vi "Seg1_Charging_Limit_current.vi"(0 "VISA Refnum in":refnum<visa-resource-name>, 1 "Value":string, 3 "Data Log Period (0.1 s)":dbl=1.0 format="%#_13g", 5 "Set Voltge(V)":dbl=4.35 format="%_3f", 7 "Log?":bool, 9 "Charge Current (A)":dbl=0.06 format="%#_13g", 11 "error in (no error)":errorcluster {"code" format="%.0x"}, 12 "Numeric":i32, 14 "Number of cycles":i32) -> (4 "VISA Refnum out":refnum<visa-resource-name>, 6 "String":string, 8 "File Name Out":string, 10 "String 2":string, 15 "error out":errorcluster)   [LabVIEW 2015]
uses:
  <instrlib>/Agilent N6700 Series/Agilent N6700 Series.lvlib
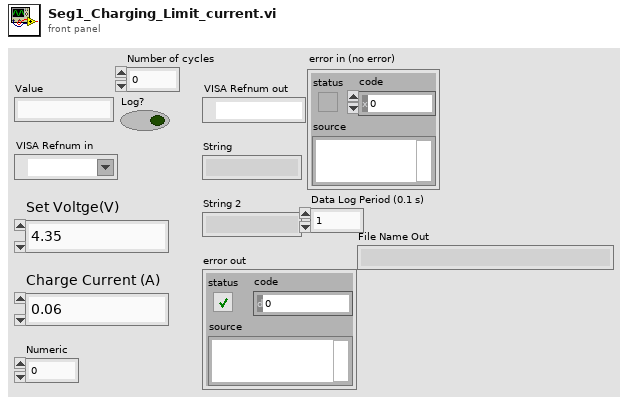
[diagram p1: front panel]
types:
  T1 = enum16{"2 Quad Power Supply", "Unipower Supply", "CC Load", "CV Load", "VM", "CM"}
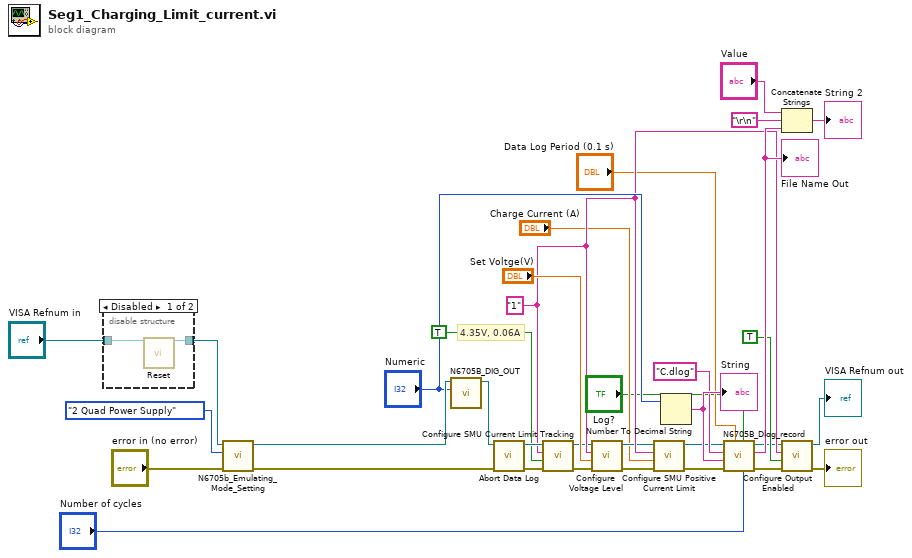
[diagram p0: block diagram]
diagram:
  w21 = "1" ("Channel Name (1)")
  # "4.35V, 0.06A"
  n1 = disable-structure shown="Disabled" {
    disable-tunnel: "VISA Refnum in" -> [w36 w37]
    disable-tunnel: [w35 w37] -> w30
    frame Disabled {
      n2 = call <instrlib>:"Reset.vi"("VISA resource name"=w36) -> ("VISA resource name out"=w35:refnum<visa-resource-name>)  [unwired: 13 in, 1 out]
    }
    frame Enabled {
    }
  }
  n3 = call "N6705b_Emulating_Mode_Setting.vi"("error in (no error)"="error in (no error)", "Mode"=T1."2 Quad Power Supply", "VISA resource name"=w30) -> ("error out"=w1:errorcluster, "VISA resource name out"=w33:refnum<visa-resource-name>)  [unwired: 7 in]
  n4 = call "N6705B_DIG_OUT.vi"("DUT_1_4"="Numeric", "VISA Refnum in"=w33) -> ("VISA Refnum out"=w34:refnum<visa-resource-name>)  [unwired: 8 in, 1 out]
  n5 = call <instrlib>:"Abort Data Log.vi"("error in (no error)"=w1, "VISA resource name"=w34) -> ("error out"=w23:errorcluster, "VISA resource name out"=w22:refnum<visa-resource-name>)  [unwired: 8 in]
  n6 = call <instrlib>:"Configure SMU Current Limit Tracking.vi"("error in (no error)"=w23, "Enable Current Limit Tracking (False)"=TRUE, "Channel Name (1)"=w21, "VISA resource name"=w22) -> ("error out"=w9:errorcluster, "VISA resource name out"=w8:refnum<visa-resource-name>)  [unwired: 6 in]
  n7 = call <instrlib>:"Configure Voltage Level.vi"("error in (no error)"=w9, "Level  (0.0 volts)"="Set Voltge(V)", "Channel Name (1)"=w21, "VISA resource name"=w8) -> ("error out"=w12:errorcluster, "VISA resource name out"=w11:refnum<visa-resource-name>)  [unwired: 6 in]
  n8 = call <instrlib>:"Configure SMU Positive Current Limit.vi"("error in (no error)"=w12, "Positive Current Limit (0.0 amps)"="Charge Current (A)", "Channel Name (1)"=w21, "VISA resource name"=w11) -> ("error out"=w15:errorcluster, "VISA resource name out"=w13:refnum<visa-resource-name>)  [unwired: 6 in]
  n9 = Number To Decimal String(number="Numeric") -> (decimal integer string=w31:string)  [unwired: 1 in]
  "String" <- w31
  n10 = call "N6705B_Dlog_record.vi"("Number of cycles"="Number of cycles", "Log?"="Log?", "Data Log Period (0.1 s)"="Data Log Period (0.1 s)", "error in (no error)"=w15, "N"=w31, "Data Log File Path (data1.dlog)"="C.dlog", "VISA resource name"=w13) -> ("error out"=w16:errorcluster, "File Name Out"=w27:string, "VISA resource name out"=w17:refnum<visa-resource-name>)  [unwired: 2 in]
  "File Name Out" <- w27
  n11 = Concatenate Strings("Value", "\r\n", w27) -> (→"String 2":string)
  n12 = call <instrlib>:"Configure Output Enabled.vi"("error in (no error)"=w16, "Enable Output (False)"=TRUE, "Channel Name (1)"=w21, "VISA resource name"=w17) -> ("error out"=→"error out":errorcluster, "VISA resource name out"=→"VISA Refnum out":refnum<visa-resource-name>)  [unwired: 6 in]
